vi "PathLoadDisplay.vi"(0 "Drive Command Strings":string[](array[string]), 1 "Drive Parameter Strings":string[](array[string]), 9 "Autonomous Path Suffix":string) -> (14 "Path X Coordinates (in)":dbl[](array[numeric]), 15 "Path Y Coordinates (in)":dbl[](array[numeric]))   [LabVIEW 2020]
uses:
  SafeParser_String.vi
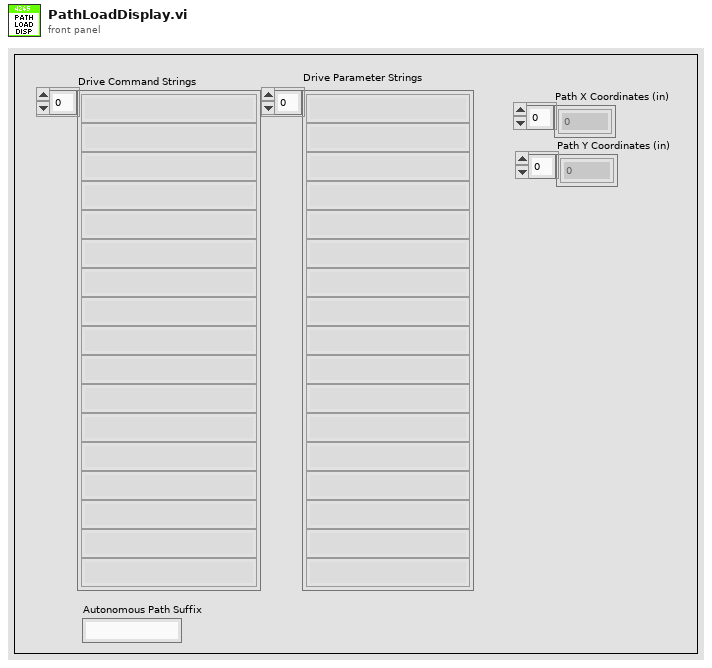
[diagram p1: front panel]
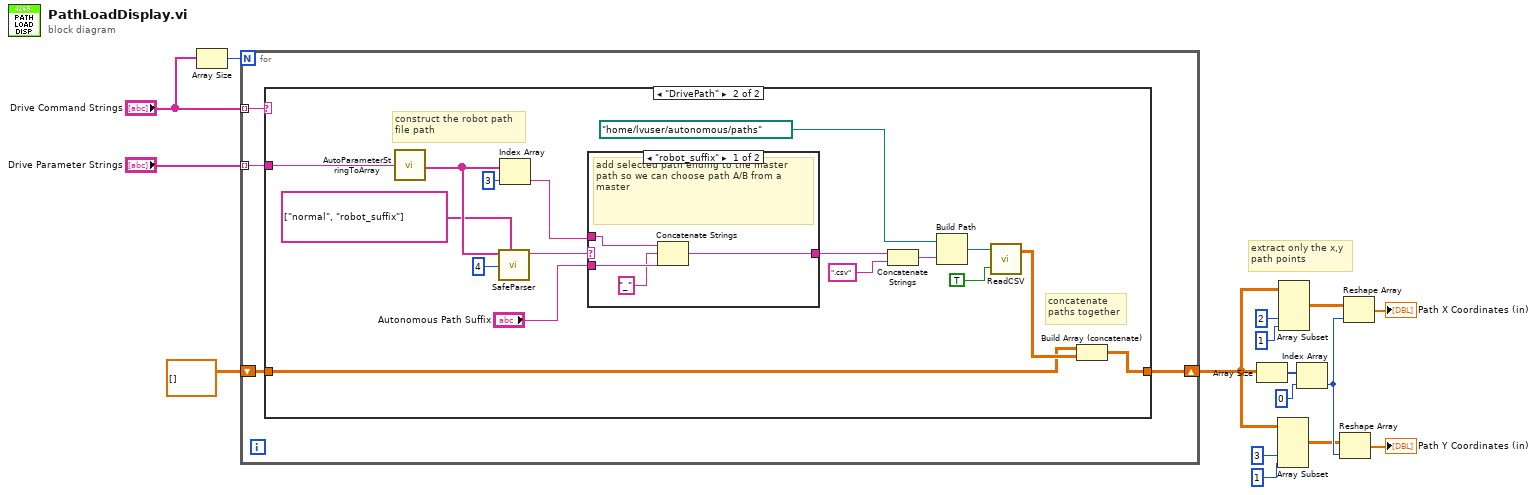
[diagram p0: block diagram]
diagram:
  # "extract only the x,y\npath points"
  n1 = Array Size(array="Drive Command Strings") -> (size(s)=w15:i32)
  n2 = for {
    N: w15 -> [_]
    tunnel: "Drive Command Strings" -> [w20] mode=indexing
    tunnel: "Drive Parameter Strings" -> [w19] mode=indexing
    shift-right: [w17] -> w3
    shift-left: dbl[][] [] ("Data (index by row)") -> [w18]
    n3 = case shown="\"DrivePath\"" w20 {
      tunnel: w19 -> [_ w26]
      tunnel: w18 -> [w21 w24]
      tunnel: [w21 w23] -> w17
      frame "Default", Default {
      }
      frame "DrivePath" {
        # "construct the robot path\nfile path"
        # "concatenate\npaths together"
        n4 = call "AutoParameterStringToArray.vi"("Parameter String"=w26) -> ("Parsed Parameters"=w37:string[])
        n5 = call-poly "SafeParser.vi"("Allowed Values"=string[] ["normal", "robot_suffix"], "Array Index"=4, "String Array"=w37) -> ("Typecast Value"=w36:string)  [unwired: 7 in, 1 out]
        n6 = Index Array(array=w37, index=3) -> (element=w34:string)
        n7 = case shown="\"robot_suffix\"" w36 {
          tunnel: w34 -> [w42 w43]
          tunnel: [w41 w43] -> w35
          tunnel: "Autonomous Path Suffix" -> [w40 _]
          frame "robot_suffix" {
            # "add selected path ending to the master \npath so we can choose path A/B from a master"
            n8 = Concatenate Strings(w42, "_" ("string"), w40) -> (w41:string)
          }
          frame "normal", Default {
          }
        }
        n9 = Concatenate Strings(w35, ".csv" ("string")) -> (w33:string)
        n10 = Build Path(base path=path "/home/lvuser/autonomous/paths" ("path"), name or relative path=w33) -> (appended path=w32:path)
        n11 = call "ReadCSV.vi"("Reinit"=TRUE, "File Path (.csv)"=w32) -> ("Data (index by row)"=w25:dbl[][])  [unwired: 1 out]
        n12 = Build Array (concatenate)(w24, w25) -> (w23:dbl[][])
      }
    }
  }
  n13 = Array Size(array=w3) -> (size(s)=w12:i32[])
  n14 = Array Subset(array=w3, index (col)=3 ("index"), length (col)=1 ("length")) -> (w10:dbl[][])  [unwired: 2 in]
  n15 = Array Subset(array=w3, index (col)=2 ("index"), length (col)=1 ("length")) -> (w11:dbl[][])  [unwired: 2 in]
  n16 = Index Array(array=w12, index=0) -> (element=w13:i32)
  n17 = Reshape Array(w10, w13) -> (→"Path Y Coordinates (in)":dbl[])
  n18 = Reshape Array(w11, w13) -> (→"Path X Coordinates (in)":dbl[])
